vi "Get Debug Mode.vi"(8 "error in (no error)":errorcluster, 11 "SMO":refnum<class "SMO.lvclass">) -> (0 "error out":errorcluster, 2 "Behavior":T1, 3 "SMO out":refnum<class "SMO.lvclass">)   [LabVIEW 2019, in "Debug.lvlib"]
uses:
  Debug.lvlib
  <vilib>/JKI/JKI SMO/SMO/SMO.lvclass
  subsystems/Attribute.Debug/DebugBehavior.ctl
  subsystems/Attribute.Debug/Attribute.Debug.lvclass/Attribute.Debug.ctl
  subsystems/SMO.Mediator/SMO.Mediator.lvclass
  subsystems/Attribute.Debug/Attribute.Debug.lvclass
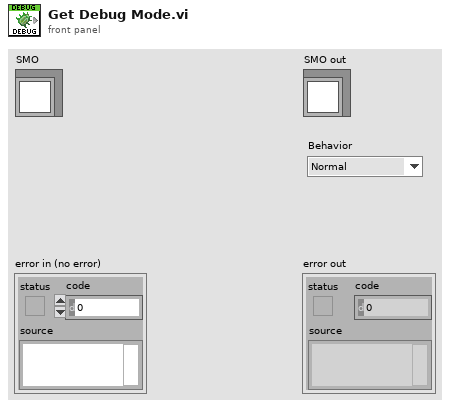
[diagram p1: front panel]
types:
  T1 = typedef "Debug.lvlib/Attribute.Debug.lvclass/DebugBehavior.ctl" = enum16{"Normal", "Debug"}
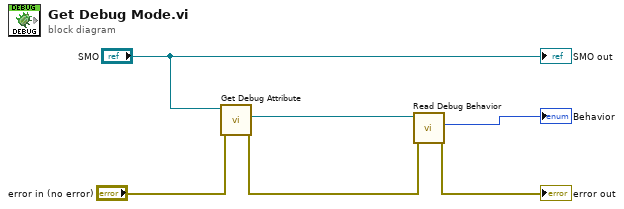
[diagram p0: block diagram]
diagram:
  n1 = call "Get Debug Attribute.vi"("error in (no error)"="error in (no error)", "SMO"="SMO") -> ("error out"=w3:errorcluster, "Attribute.Debug"=w4:refnum<class "Attribute.Debug.lvclass">)  [unwired: 7 in, 1 out]
  n2 = call "Read Debug Behavior.vi"("error in (no error)"=w3, "Attribute.Debug in"=w4) -> ("error out"=→"error out":errorcluster, "Behavior"=→"Behavior":T1)  [unwired: 7 in, 1 out]
  "SMO out" <- "SMO"
